vi "Orb_Check.vi"(0 "error in (no error)":errorcluster) -> (3 "error out":errorcluster, 6 "Orb Running ?":bool)   [LabVIEW 2009]
uses:
  Instance           2 17Saved   Orb_Check .vi
  Orb_Global.vi
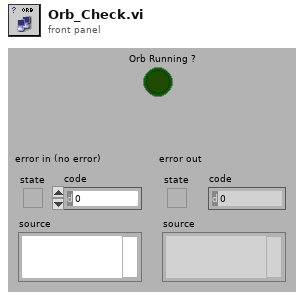
[diagram p1: front panel]
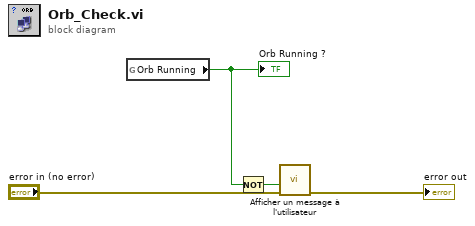
[diagram p0: block diagram]
diagram:
  n1 = global read "Orb_Global.vi" "Orb Running"() -> (w2:bool)
  "Orb Running ?" <- w2
  n2 = Not(x=w2) -> (.not. x?=w1:bool)
  n3 = call "Afficher un message à l'utilisateur"("error in (no error)"="error in (no error)", "Enable"=w1) -> ("error out"=→"error out":errorcluster)  [unwired: 1 in, 8 out]
